vi "TH_RS232_Read.vi"(0 "COMhandles In":refnum<visa-resource-name>[](array[refnum]), 3 "error in array":errorcluster[](array[cluster])) -> (4 "NewValues Out":bool[](array[boolean]), 5 "COMhandles Out":refnum<visa-resource-name>[](array[refnum]), 6 "Temperatures":dbl[](array[numeric])=[nan, nan, nan] format="%.2f", 7 "Humidities":dbl[](array[numeric])=[nan, nan, nan] format="%.2f", 8 "error out array":errorcluster[](array[cluster]))   [LabVIEW 2020]
panel:
  out "LastTime":ext[](array[numeric]) format="%.2f"
  out "RawString":string[](array[string])
  out "Bytes at Port":i32[](array[numeric])
  # "! These three must be initiated to display NaN instead of 0.0 !"
  # "Local Variables"
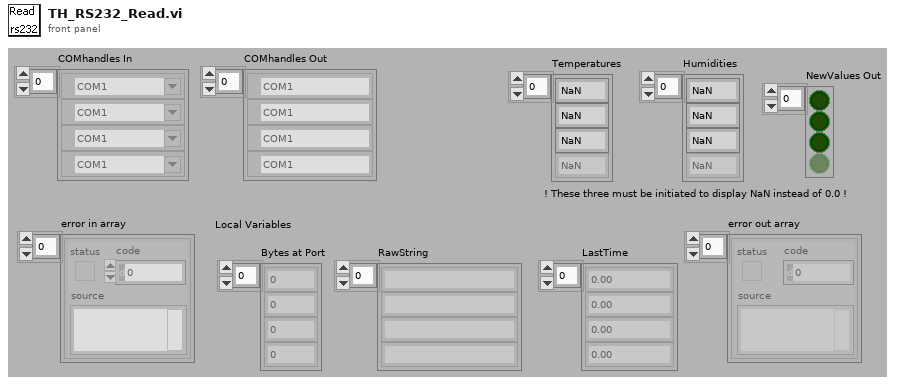
[diagram p1: front panel]
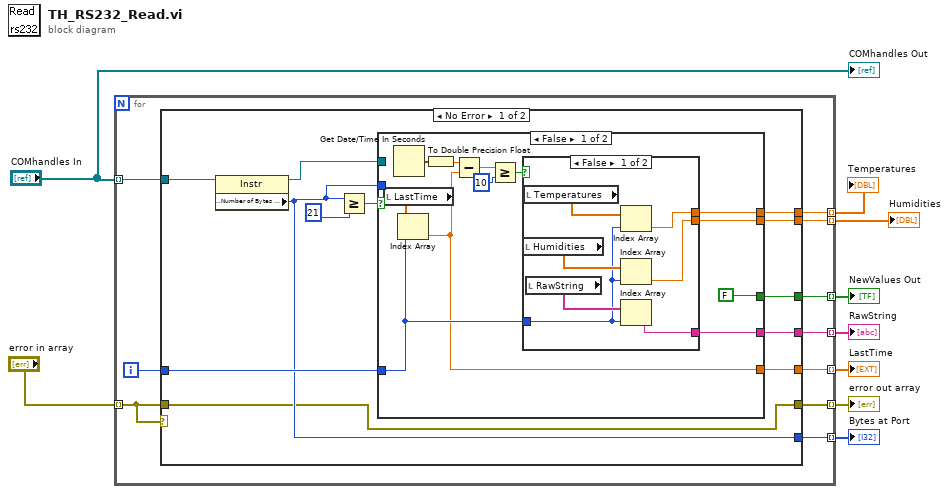
[diagram p0: block diagram]
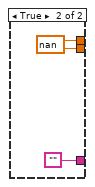
[diagram p2: hidden frame]
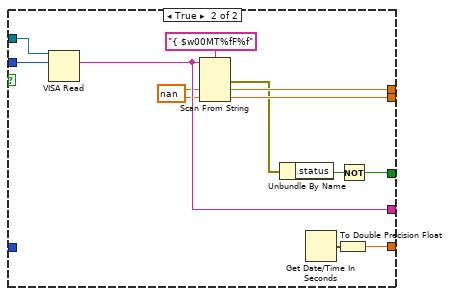
[diagram p3: hidden frame]
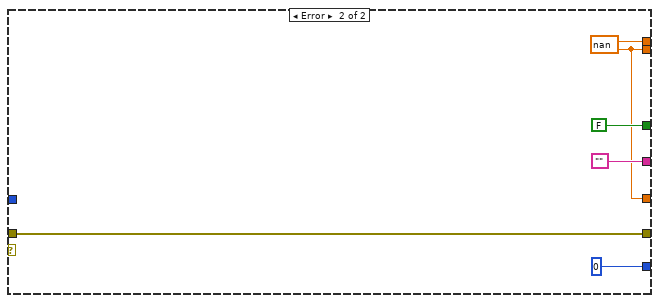
[diagram p4: hidden frame]
diagram:
  n1 = for {
    tunnel: "COMhandles In" -> [w19] mode=indexing
    tunnel: [w18] -> w7 mode=indexing
    tunnel: [w17] -> w6 mode=indexing
    tunnel: [w15] -> w5 mode=indexing
    tunnel: [w14] -> w4 mode=indexing
    tunnel: [w13] -> w3 mode=indexing
    tunnel: [w12] -> w9 mode=indexing
    tunnel: "error in array" -> [w11] mode=indexing
    tunnel: [w10] -> w1 mode=indexing
    i -> [w16]
    n2 = case shown="No Error" w11 {
      tunnel: w19 -> [w30 _]
      tunnel: [w28 w65] -> w18
      tunnel: [w27 w65] -> w17
      tunnel: w16 -> [w26 _]
      tunnel: [w25 0] -> w15
      tunnel: [w24 ""] -> w14
      tunnel: [w23 FALSE] -> w13
      tunnel: [w20 w69] -> w12
      tunnel: w11 -> [w20 w69]
      tunnel: [w21 w65] -> w10
      frame No Error {
        n3 = property class="Instr"(reference=w30) -> (reference out=w22:refnum<visa-resource-name>, "Serial Settings:Number of Bytes at Serial Port"=w25:u32)  [unwired: 1 in, 1 out]
        n4 = Greater Or Equal?(x=w25, y=u32 21) -> (x >= y?=w31:bool)
        n5 = case shown="False" w31 {
          tunnel: w22 -> [_ w64]
          tunnel: w25 -> [_ w63]
          tunnel: [w43 w61] -> w28
          tunnel: [w42 w60] -> w27
          tunnel: w26 -> [w39 _]
          tunnel: [w41 w59] -> w24
          tunnel: [FALSE w57] -> w23
          tunnel: [w33 w55] -> w21
          frame False {
            n6 = local read "LastTime"() -> (w37:ext[])
            n7 = Get Date/Time In Seconds() -> (seconds since 1Jan1904=w32:timestamp)
            n8 = Index Array(array=w37, index=w39) -> (element=w33:ext)
            n9 = To Double Precision Float(number=w32) -> (double precision float=w38:dbl)
            n10 = Subtract(x=w38, y=w33) -> (x-y=w36:ext)
            n11 = Greater Or Equal?(x=w36, y=u32 10) -> (x >= y?=w34:bool)
            n12 = case shown="False" w34 {
              tunnel: [w48 w52] -> w43
              tunnel: [w47 w52] -> w42
              tunnel: [w45 ""] -> w41
              tunnel: w39 -> [w44 _]
              frame False {
                n13 = local read "Humidities"() -> (w49:dbl[])
                n14 = local read "Temperatures"() -> (w50:dbl[])
                n15 = local read "RawString"() -> (w46:string[])
                n16 = Index Array(array=w50, index=w44) -> (element=w48:dbl)
                n17 = Index Array(array=w49, index=w44) -> (element=w47:dbl)
                n18 = Index Array(array=w46, index=w44) -> (element=w45:string)
              }
              frame True {
                w52 = nan
              }
            }
          }
          frame True {
            w56 = nan
            n19 = VISA Read(VISA resource name=w64, byte count=w63) -> (read buffer=w59:string)  [unwired: 1 in, 3 out]
            n20 = Scan From String(format string="{ $w00MT%fF%f", input string=w59, default 1=w56, default 2=w56) -> (error out=w54:errorcluster, output 1=w61:dbl, output 2=w60:dbl)  [unwired: 2 in, 2 out]
            n21 = Unbundle By Name(w54) -> ("status"=w58:bool)
            n22 = Get Date/Time In Seconds() -> (seconds since 1Jan1904=w53:timestamp)
            n23 = To Double Precision Float(number=w53) -> (double precision float=w55:dbl)
            n24 = Not(x=w58) -> (.not. x?=w57:bool)
          }
        }
      }
      frame Error {
        w65 = nan
      }
    }
  }
  "error out array" <- w9
  "Temperatures" <- w7
  "Humidities" <- w6
  "Bytes at Port" <- w5
  "RawString" <- w4
  "NewValues Out" <- w3
  "LastTime" <- w1
  "COMhandles Out" <- "COMhandles In"
